vi "GET.vi"(6 "timeout":i32=10000, 7 "output file":path, 8 "error in":errorcluster, 10 "url":string, 11 "session in":refnum<class "Session.lvclass">) -> (0 "error out":errorcluster, 1 "body":string, 2 "headers":string, 3 "session out":refnum<class "Session.lvclass">, 4 "status code":u32)   [LabVIEW 2024, in "lib_NI_Advanced HTTP Client.lvlib" / "Session.lvclass"]
doc: "Sends a web request that returns header and body data from a server, web page, or web service. This VI uses the GET HTTP method and does not submit any data to the server."
uses:
  Session.lvclass
  Session.lvclass/Session.ctl
  lvwebclient_64.dll
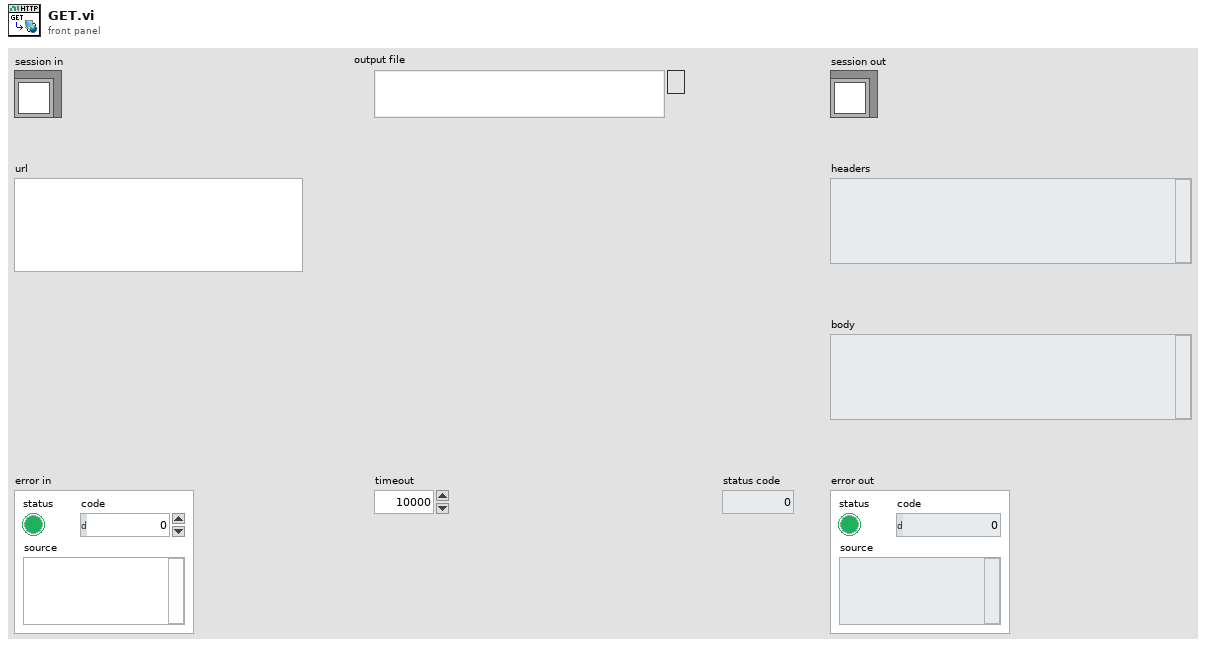
[diagram p1: front panel]
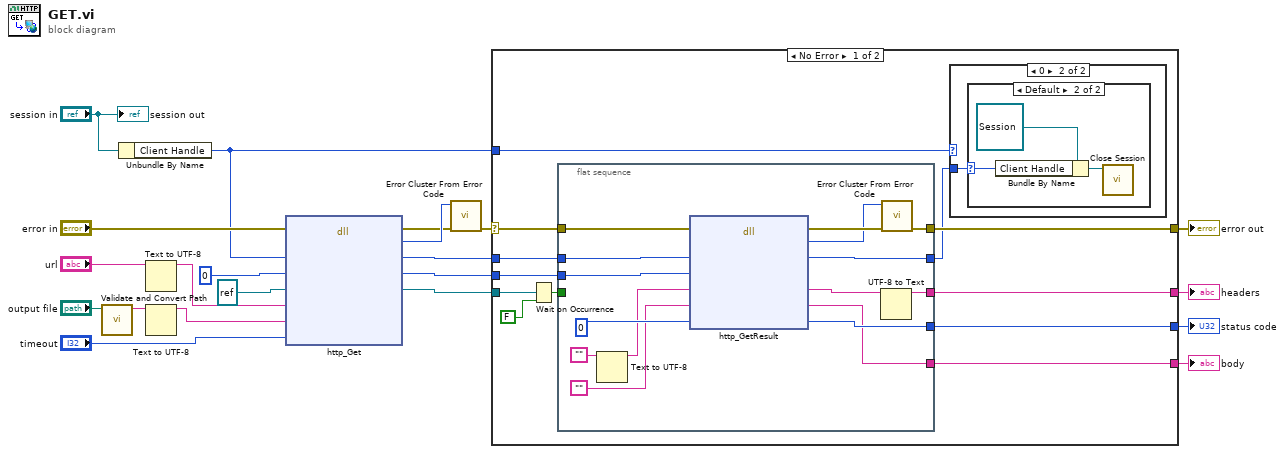
[diagram p0: block diagram]
diagram:
  n1 = call "Validate and Convert Path.vi"("path"="output file") -> ("validated path as string"=w1:string)  [unwired: 10 in]
  n2 = Unbundle By Name("session in") -> ("Client Handle"=w3:u32)
  n3 = Text to UTF-8(11:"url") -> (3:w15:string)  [unwired: 2 in, 1 out]
  n4 = Text to UTF-8(11:w1) -> (3:w12:string)  [unwired: 2 in, 1 out]
  n5 = dll-call lib="C:/Program Files/National Instruments/LabVIEW 2024/vi.lib/NI/Advanced HTTP Client/lvwebclient_*.*" fn="http_Get"(error in="error in", "handle"=w3, "request"=u32 0, "completeOccurrence"=refnum<k4> refnum ("occurrence"), "url"=w15, "outPath"=w12, "timeout"="timeout") -> (error out=w11:errorcluster, "return"=w19:i32, "handle"=w9:u32, "request"=w8:u32, "completeOccurrence"=w13:refnum<k4>)  [unwired: 5 in, 1 out]
  n6 = call "Error Cluster From Error Code.vi"("error in (no error)"=w11, "error code (0)"=w19) -> ("error out"=w21:errorcluster)  [unwired: 7 in]
  n7 = case shown="No Error" w21 {
    selector: w21 -> [w31 w53]
    tunnel: w13 -> [w33 _]
    tunnel: w9 -> [w30 _]
    tunnel: w8 -> [w29 _]
    tunnel: [w28 _] -> w7
    tunnel: [w27 _] -> w6
    tunnel: [w26 _] -> w5
    tunnel: [w25 w53] -> w4
    tunnel: w3 -> [w24 _]
    frame No Error {
      n8 = Wait on Occurrence(1:FALSE, 2:w33) -> (0:w32:bool)  [unwired: 1 in]
      n9 = flat-sequence {
        tunnel: w32 -> [_]
        tunnel: w31 -> [w52]
        tunnel: w30 -> [w51]
        tunnel: w29 -> [w50]
        tunnel: [w48] -> w28
        tunnel: [w44] -> w27
        tunnel: [w39] -> w26
        tunnel: [w43] -> w25
        tunnel: [w42] -> w23
        frame #0 {
          n10 = Text to UTF-8(11:"") -> (3:w40:string)  [unwired: 2 in, 1 out]
          n11 = dll-call lib="C:/Program Files/National Instruments/LabVIEW 2024/vi.lib/NI/Advanced HTTP Client/lvwebclient_*.*" fn="http_GetResult"(error in=w52, "handle"=w51, "request"=w50, "returnHeader"=w40, "returnBody"="", "httpStatus"=u32 0) -> (error out=w47:errorcluster, "return"=w46:i32, "handle"=w42:u32, "returnHeader"=w45:string, "returnBody"=w39:string, "httpStatus"=w48:u32)  [unwired: 3 in, 1 out]
          n12 = UTF-8 to Text(11:w45) -> (3:w44:string)  [unwired: 2 in, 1 out]
          n13 = call "Error Cluster From Error Code.vi"("error in (no error)"=w47, "error code (0)"=w46) -> ("error out"=w43:errorcluster)  [unwired: 7 in]
        }
      }
      n14 = case shown="0" w24 {
        tunnel: w23 -> [_ w34]
        frame Default {
        }
        frame 0 {
          n15 = case shown="Default" w34 {
            selector: w34 -> [_ w37]
            frame 0 {
            }
            frame Default {
              n16 = Bundle By Name(cluster=refnum<class "Session.lvclass"> refnum ("NI_Advanced HTTP Client.lvlib:Session.lvclass"), "Client Handle"=w37) -> (w36:refnum<class "Session.lvclass">)
              n17 = call "Close Session.vi"("session"=w36) -> ()  [unwired: 10 in, 1 out]
            }
          }
        }
      }
    }
    frame Error {
    }
  }
  "error out" <- w4
  "headers" <- w6
  "body" <- w5
  "status code" <- w7
  "session out" <- "session in"
